vi "AddGlyphtoGManager.vi"(8 "error in":errorcluster, 10 "glyph manager":T1, 11 "NISE_CEF_serializable node in":refnum<class "NISE_CEF_serializable node.lvclass">) -> (0 "error out":errorcluster, 2 "glyph manager out":T1, 3 "NISE_CEF_serializable node out":refnum<class "NISE_CEF_serializable node.lvclass">)   [LabVIEW 2013, in "NISE_CEF_serializable node.lvclass"]
uses:
  NISE_CEF_serializable node.lvclass
  glyph manager/glyph manager.ctl
  <vilib>/picture/picture.llb/imagedata.ctl
  Node/NISE_CEF_Node.lvclass
  glyph manager/glyph manager.lvlib
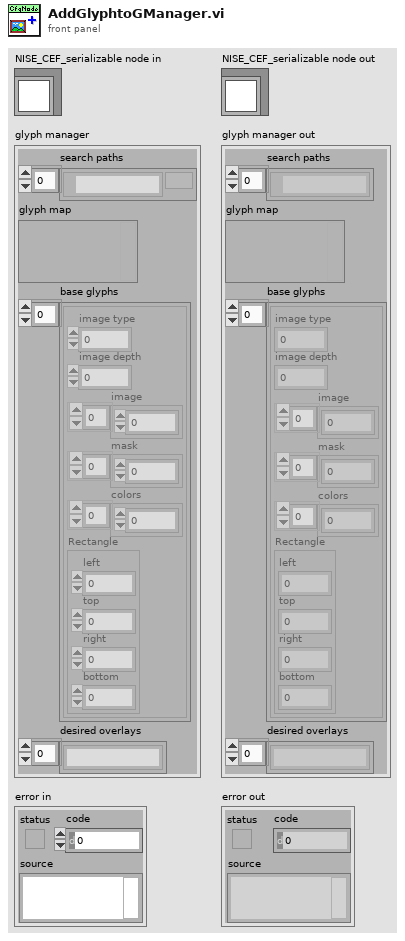
[diagram p1: front panel]
types:
  T1 = typedef "glyph manager.lvlib/glyph manager.ctl" = cluster{"search paths":path[], "glyph map":variant, "base glyphs":T2[], "desired overlays":string[]}
  T2 = typedef "imagedata.ctl" = cluster{"image type":i32, "image depth":i32, "image":u8[], "mask":u8[], "colors":u32[], "Rectangle":cluster{"left":i16, "top":i16, "right":i16, "bottom":i16}}
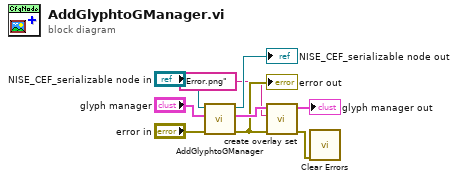
[diagram p0: block diagram]
diagram:
  n1 = call-parent "AddGlyphtoGManager.vi"("error in"="error in", "glyph manager"="glyph manager", "NISE_CEF_Node in"="NISE_CEF_serializable node in") -> ("error out"=w3:errorcluster, "glyph manager out"=w5:T1, "NISE_CEF_Node out"=→"NISE_CEF_serializable node out":refnum<class "NISE_CEF_serializable node.lvclass">)  [unwired: 6 in]
  "error out" <- w3
  n2 = call "create overlay set.vi"("error in"=w3, "overlay glyph"="Error.png", "glyph manager in"=w5) -> ("error out"=w2:errorcluster, "glyph manager out"=→"glyph manager out":T1)  [unwired: 7 in]
  n3 = call <vilib>:"Clear Errors.vi"("error in (no error)"=w2) -> ()  [unwired: 6 in, 1 out]
